vi "Hybrid PS Set Setpoint.vi"(0 "Setpoint":dbl format="%.2f", 1 "Change it":bool, 2 "VI Refnum":refnum<vi>) -> ()   [LabVIEW 2020]
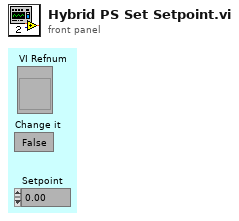
[diagram p1: front panel]
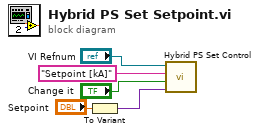
[diagram p0: block diagram]
diagram:
  n1 = To Variant(anything="Setpoint") -> (Variant=w2:variant)
  n2 = call "Hybrid PS Set Control.vi"("Value"=w2, "Change it"="Change it", "Control Name"="Setpoint [kA]" ("y"), "VI Refnum"="VI Refnum") -> ()
